vi "SetSystemDefinitionPropertyValueFromString.vi"(8 "error in (no error)":errorcluster, 9 "value":string, 10 "property name":string, 11 "BaseNodeType in":refnum<k24>) -> (0 "error out":errorcluster, 3 "BaseNodeType out":refnum<k24>)   [LabVIEW 2015, in "VeriStandTestUtilities.lvlib"]
uses:
  VeriStandTestUtilities.lvlib
  SetSystemDefinitionPropertyValue_Bool.vi
  SetSystemDefinitionPropertyValue_U64.vi
  SetSystemDefinitionPropertyValue_U32.vi
  SetSystemDefinitionPropertyValue_U16.vi
  SetSystemDefinitionPropertyValue_I64.vi
  SetSystemDefinitionPropertyValue_I32.vi
  SetSystemDefinitionPropertyValue_I16.vi
  SetSystemDefinitionPropertyValue_Double.vi
  SetSystemDefinitionPropertyValue_String.vi
  NationalInstruments.VeriStand.SystemStorage
  SetSystemDefinitionPropertyValue_BinaryString.vi
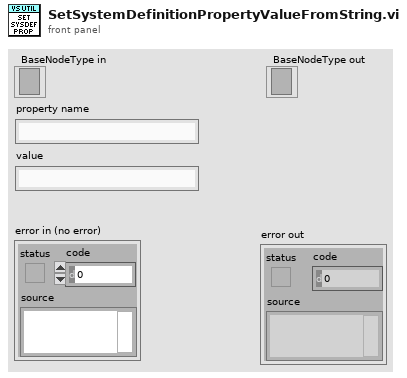
[diagram p1: front panel]
types:
  T1 = typedef "VeriStandTestUtilities.lvlib/SystemDefinitionPropertyType.ctl" = enum16{"K_STRING", "K_BOOL", "K_I32", "K_U32", "K_DOUBLE", "K_U64", "K_VARIANT", "K_DEPENDENTFILE", "K_DEPENDENTNODE", "K_DATASOURCENODE", "K_U16", "K_DBLARR", "K_U32ARR", "K_I32ARR", "K_STRINGARR", "K_DICTIONARY", "K_DICTIONARYARR", "K_BINARYSTRING", "K_I16", "K_I64", "K_BOOLARR", "K_U64ARR", "K_U16ARR", "K_I64ARR", "K_I16ARR"}
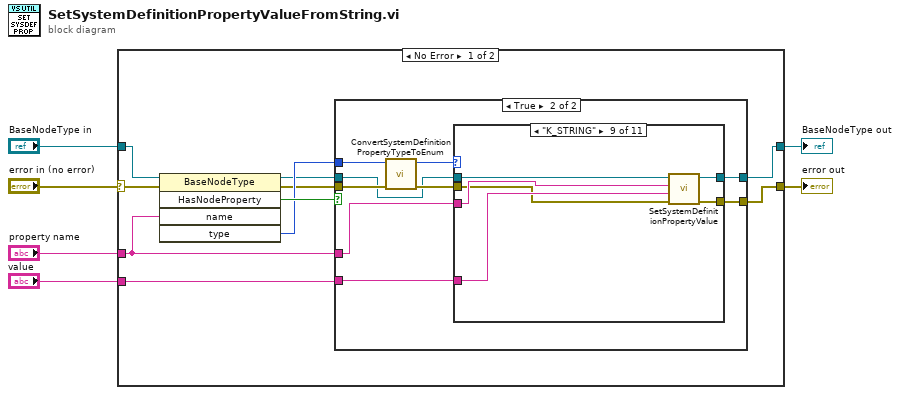
[diagram p0: block diagram]
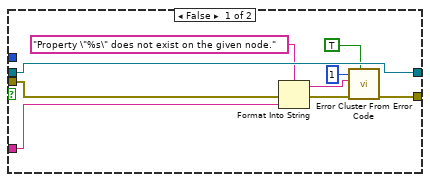
[diagram p2: hidden frame]
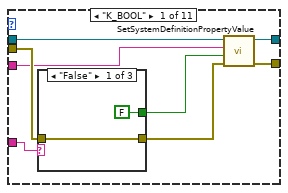
[diagram p3: hidden frame]
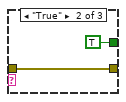
[diagram p4: hidden frame]
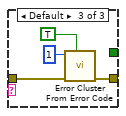
[diagram p5: hidden frame]
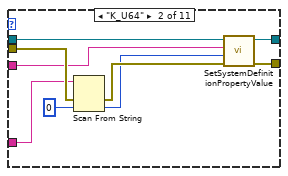
[diagram p6: hidden frame]
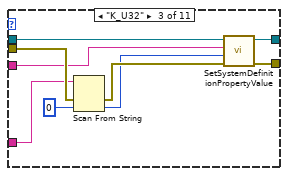
[diagram p7: hidden frame]
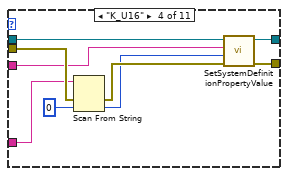
[diagram p8: hidden frame]
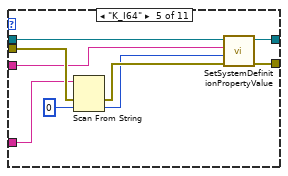
[diagram p9: hidden frame]
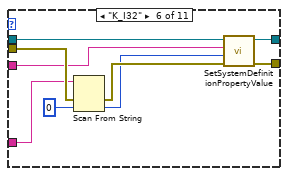
[diagram p10: hidden frame]
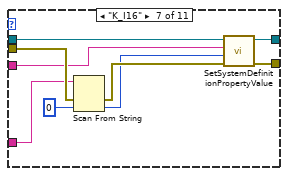
[diagram p11: hidden frame]
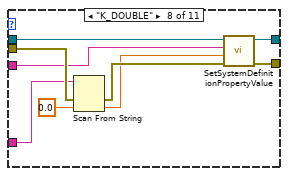
[diagram p12: hidden frame]
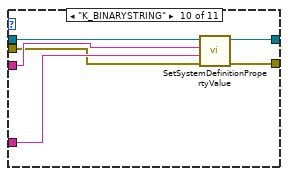
[diagram p13: hidden frame]
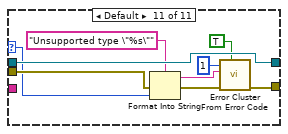
[diagram p14: hidden frame]
diagram:
  n1 = case shown="No Error" "error in (no error)" {
    selector: "error in (no error)" -> [w16 w136]
    tunnel: [w11 w136] -> w6
    tunnel: [w10 w135] -> w4
    tunnel: "BaseNodeType in" -> [w9 w135]
    tunnel: "property name" -> [w8 _]
    tunnel: "value" -> [w7 _]
    frame No Error {
      n2 = invoke class="BaseNodeType" method="HasNodeProperty"(reference=w9, error in=w16, "name"=w8) -> (reference out=w12:refnum<k24>, error out=w13:errorcluster, "HasNodeProperty"=w15:bool, "type"=w14:i32)  [unwired: 2 in, 1 out]
      n3 = case shown="True" w15 {
        tunnel: w14 -> [_ w34]
        tunnel: w13 -> [w22 w32]
        tunnel: w12 -> [w25 w30]
        tunnel: [w21 w29] -> w11
        tunnel: [w25 w28] -> w10
        tunnel: w8 -> [w23 w27]
        tunnel: w7 -> [_ w26]
        frame False {
          n4 = Format Into String(format string="Property \"%s\" does not exist on the given node.", error in=w22, w23) -> (resulting string=w19:string, error out=w20:errorcluster)  [unwired: 1 in]
          n5 = call <vilib>:"Error Cluster From Error Code.vi"("show call chain? (False)"=TRUE, "error in (no error)"=w20, "error message (\"\")"=w19, "error code (0)"=1) -> ("error out"=w21:errorcluster)  [unwired: 5 in]
        }
        frame True {
          n6 = call "ConvertSystemDefinitionPropertyTypeToEnum.vi"("error in (no error)"=w32, "type"=w34) -> ("error out"=w31:errorcluster, "type"=w33:T1)  [unwired: 8 in]
          n7 = case shown="\"K_STRING\"" w33 {
            selector: w33 -> [_ _ _ _ _ _ _ _ _ _ w127]
            tunnel: w31 -> [w38 w59 w68 w77 w86 w95 w104 w113 w114 w120 w128]
            tunnel: w30 -> [w42 w56 w65 w74 w83 w92 w101 w110 w119 w125 w134]
            tunnel: [w41 w54 w63 w72 w81 w90 w99 w108 w117 w123 w129] -> w29
            tunnel: [w40 w55 w64 w73 w82 w91 w100 w109 w118 w124 w134] -> w28
            tunnel: w27 -> [w35 w52 w61 w70 w79 w88 w97 w106 w116 w122 _]
            tunnel: w26 -> [w39 w57 w66 w75 w84 w93 w102 w111 w115 w121 _]
            frame "K_BOOL" {
              n8 = case shown="\"False\"" w39 {
                tunnel: [FALSE TRUE _] -> w36
                tunnel: w38 -> [w43 w45 w49]
                tunnel: [w43 w45 w50] -> w37
                frame "False" {
                }
                frame "True" {
                }
                frame Default {
                  n9 = call <vilib>:"Error Cluster From Error Code.vi"("show call chain? (False)"=TRUE, "error in (no error)"=w49, "error code (0)"=1) -> ("error out"=w50:errorcluster)  [unwired: 6 in]
                }
              }
              n10 = call-poly "SetSystemDefinitionPropertyValue.vi"("error in (no error)"=w37, "value"=w36, "property name"=w35, "BaseNodeType in"=w42) -> ("error out"=w41:errorcluster, "BaseNodeType out"=w40:refnum<k24>)  [unwired: 6 in]
            }
            frame "K_U64" {
              n11 = Scan From String(input string=w57, error in=w59, default 1=u64 0) -> (error out=w53:errorcluster, output 1=w51:u64)  [unwired: 2 in, 2 out]
              n12 = call-poly "SetSystemDefinitionPropertyValue.vi"("error in (no error)"=w53, "value"=w51, "property name"=w52, "BaseNodeType in"=w56) -> ("error out"=w54:errorcluster, "BaseNodeType out"=w55:refnum<k24>)  [unwired: 6 in]
            }
            frame "K_U32" {
              n13 = Scan From String(input string=w66, error in=w68, default 1=u32 0) -> (error out=w62:errorcluster, output 1=w60:u32)  [unwired: 2 in, 2 out]
              n14 = call-poly "SetSystemDefinitionPropertyValue.vi"("error in (no error)"=w62, "value"=w60, "property name"=w61, "BaseNodeType in"=w65) -> ("error out"=w63:errorcluster, "BaseNodeType out"=w64:refnum<k24>)  [unwired: 6 in]
            }
            frame "K_U16" {
              n15 = Scan From String(input string=w75, error in=w77, default 1=u16 0) -> (error out=w71:errorcluster, output 1=w69:u16)  [unwired: 2 in, 2 out]
              n16 = call-poly "SetSystemDefinitionPropertyValue.vi"("error in (no error)"=w71, "value"=w69, "property name"=w70, "BaseNodeType in"=w74) -> ("error out"=w72:errorcluster, "BaseNodeType out"=w73:refnum<k24>)  [unwired: 6 in]
            }
            frame "K_I64" {
              n17 = Scan From String(input string=w84, error in=w86, default 1=i64 0) -> (error out=w80:errorcluster, output 1=w78:i64)  [unwired: 2 in, 2 out]
              n18 = call-poly "SetSystemDefinitionPropertyValue.vi"("error in (no error)"=w80, "value"=w78, "property name"=w79, "BaseNodeType in"=w83) -> ("error out"=w81:errorcluster, "BaseNodeType out"=w82:refnum<k24>)  [unwired: 6 in]
            }
            frame "K_I32" {
              n19 = Scan From String(input string=w93, error in=w95, default 1=0) -> (error out=w89:errorcluster, output 1=w87:i32)  [unwired: 2 in, 2 out]
              n20 = call-poly "SetSystemDefinitionPropertyValue.vi"("error in (no error)"=w89, "value"=w87, "property name"=w88, "BaseNodeType in"=w92) -> ("error out"=w90:errorcluster, "BaseNodeType out"=w91:refnum<k24>)  [unwired: 6 in]
            }
            frame "K_I16" {
              n21 = Scan From String(input string=w102, error in=w104, default 1=i16 0) -> (error out=w98:errorcluster, output 1=w96:i16)  [unwired: 2 in, 2 out]
              n22 = call-poly "SetSystemDefinitionPropertyValue.vi"("error in (no error)"=w98, "value"=w96, "property name"=w97, "BaseNodeType in"=w101) -> ("error out"=w99:errorcluster, "BaseNodeType out"=w100:refnum<k24>)  [unwired: 6 in]
            }
            frame "K_DOUBLE" {
              n23 = Scan From String(input string=w111, error in=w113, default 1=0.0) -> (error out=w107:errorcluster, output 1=w105:dbl)  [unwired: 2 in, 2 out]
              n24 = call-poly "SetSystemDefinitionPropertyValue.vi"("error in (no error)"=w107, "value"=w105, "property name"=w106, "BaseNodeType in"=w110) -> ("error out"=w108:errorcluster, "BaseNodeType out"=w109:refnum<k24>)  [unwired: 6 in]
            }
            frame "K_STRING" {
              n25 = call-poly "SetSystemDefinitionPropertyValue.vi"("error in (no error)"=w114, "value"=w115, "property name"=w116, "BaseNodeType in"=w119) -> ("error out"=w117:errorcluster, "BaseNodeType out"=w118:refnum<k24>)  [unwired: 6 in]
            }
            frame "K_BINARYSTRING" {
              n26 = call-poly "SetSystemDefinitionPropertyValue.vi"("error in (no error)"=w120, "value"=w121, "property name"=w122, "BaseNodeType in"=w125) -> ("error out"=w123:errorcluster, "BaseNodeType out"=w124:refnum<k24>)  [unwired: 6 in]
            }
            frame Default {
              n27 = Format Into String(format string="Unsupported type \"%s\"", error in=w128, w127) -> (resulting string=w132:string, error out=w133:errorcluster)  [unwired: 1 in]
              n28 = call <vilib>:"Error Cluster From Error Code.vi"("show call chain? (False)"=TRUE, "error in (no error)"=w133, "error message (\"\")"=w132, "error code (0)"=1) -> ("error out"=w129:errorcluster)  [unwired: 5 in]
            }
          }
        }
      }
    }
    frame Error {
    }
  }
  "error out" <- w6
  "BaseNodeType out" <- w4
